vi "Normal Mode FPGA.vi"(8 "error in (no error)":errorcluster) -> (0 "error out":errorcluster)   [LabVIEW 2023, in "FPGA.lvlib"]
uses:
  FPGA.lvlib
  Internal Communication/Internal Communication.lvlib
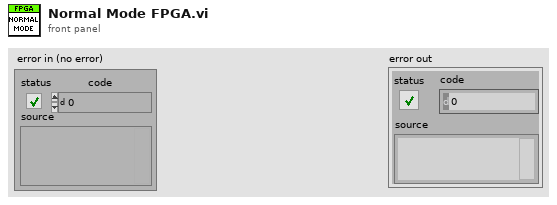
[diagram p1: front panel]
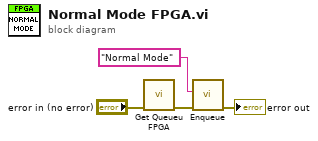
[diagram p0: block diagram]
diagram:
  n1 = call "Get Queueu FPGA.vi"("error in (no error)"="error in (no error)") -> ("error out"=w4:errorcluster)  [unwired: 9 in, 1 out]
  n2 = call "Enqueue.vi"("error in (no error)"=w4, "Command"="Normal Mode") -> ("error out"=→"error out":errorcluster)  [unwired: 8 in, 1 out]
